vi "WSVCAP SHL Host LL I2C Read.vi"(0 "Bytes to Read":u8=8, 1 "Wait Ticks":u32, 2 "Slave Address":u8, 5 "Sub Address [U8]":u8=191 format="%.0x", 7 "Socket Mask [U64]":u64=1 format="%012x", 11 "error in":errorcluster, 12 "UUT Set (0/1)":u8) -> (4 "C1:1-18 Read Data [DUT Ordered]":u8[][](array[numeric]), 6 "C2:1-18 Read Data [DUT Ordered]":u8[][](array[numeric]), 8 "C3:1-18 Read Data [DUT Ordered]":u8[][](array[numeric]), 10 "Status":u8[](array[numeric]) format="%.0x", 15 "error out":errorcluster)   [LabVIEW 2012]
uses:
  Type Defs/WSVCAP SHL Top Level Write Read State Enum.ctl
  Type Defs/WSVCAP SHL State.ctl
  Type Defs/WSVCAP SHL Transaction Enum.ctl
  Type Defs/WSVCAP SHL Top Level Control Enum.ctl
panel:
  out "Bit Array":u64[](array[numeric]) format="%.0x"
  out "Data Headers":u8[](array[numeric])=[1, 2, 3, 4, 5, 6, 7, 8, 9, 10, 11, 12, 12, 14, 15, 16]
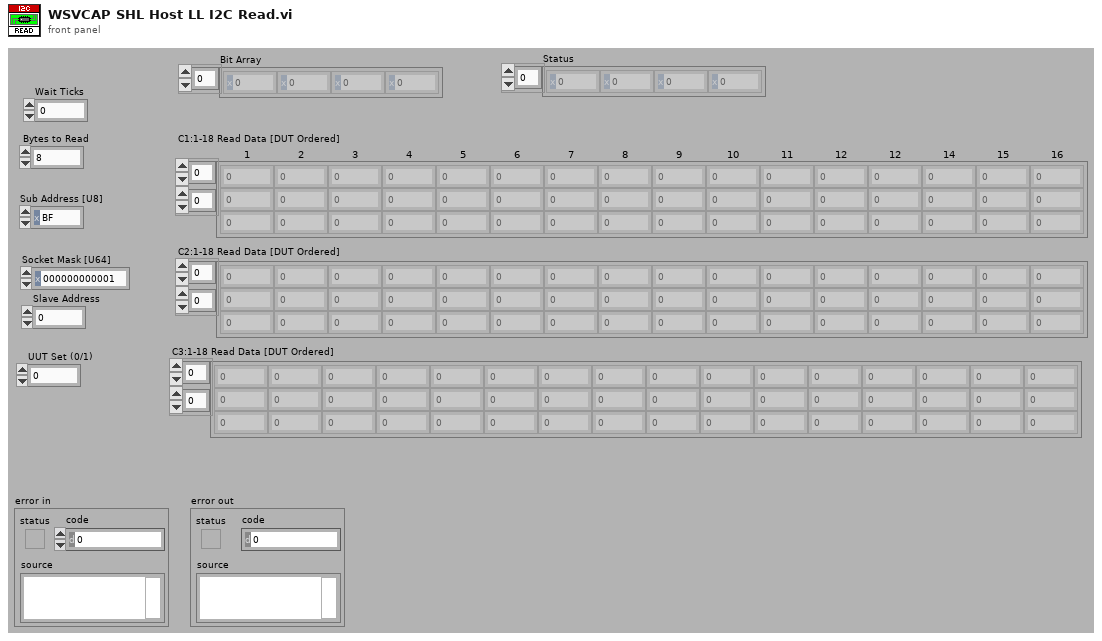
[diagram p1: front panel]
types:
  T1 = typedef "WSVCAP SHL Top Level Write Read State Enum.ctl" = enum16{"Start", "Write", "Read", "Get Status", "Wait Until Done"}
  T2 = typedef "WSVCAP SHL Transaction Enum.ctl" = enum16{"I2C-Read Data", "I2C-Write Data", "RFFE-Ext Write", "RFFE-Ext Read"}
  T3 = typedef "WSVCAP SHL Top Level Control Enum.ctl" = enum16{"Start", "Cmd", "Transaction", "Wait Ticks", "Socket Mask", "UUT Set", "Slave Address", "Sub Address", "Bytes to Write", "Bytes to Read", "Write Data", "Write Flag", "Read Data", "Read Flag", "Ack Read", "Read Status Flag", "Ack Read Status", "Status", "Cycle Count", "Stop Cycle", "Exit"}
  T4 = typedef "WSVCAP SHL State.ctl" = enum8{"Idle", "Transfer Data"}
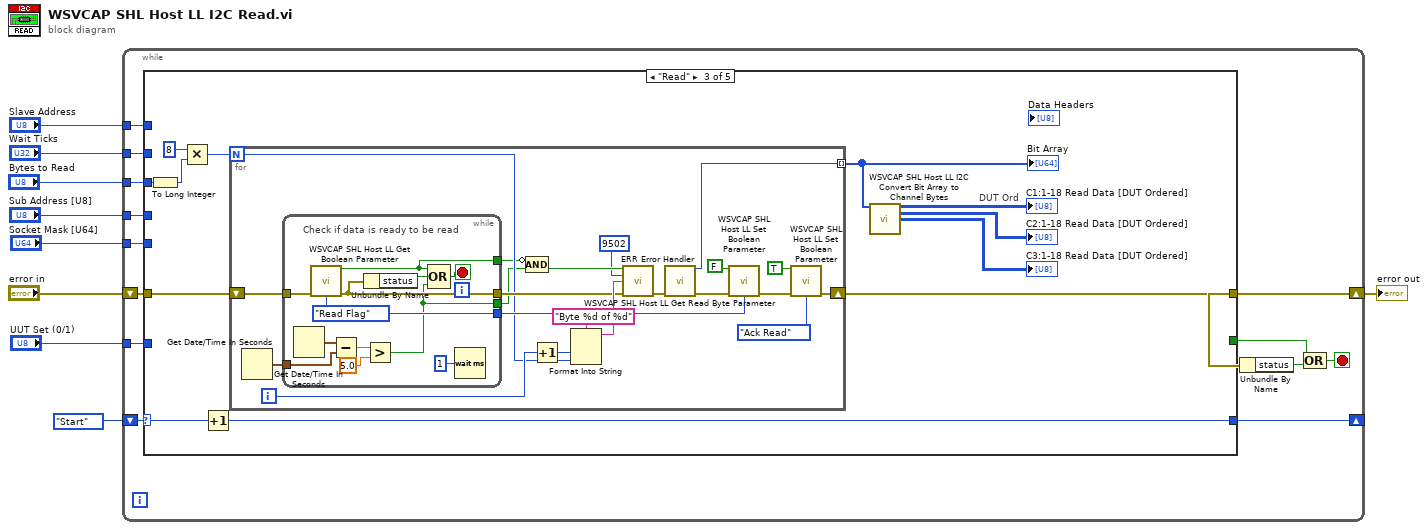
[diagram p0: block diagram]
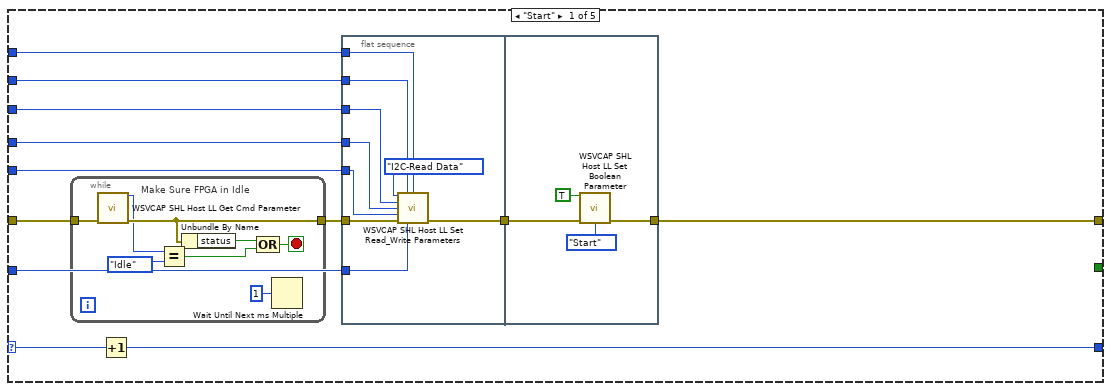
[diagram p2: hidden frame]
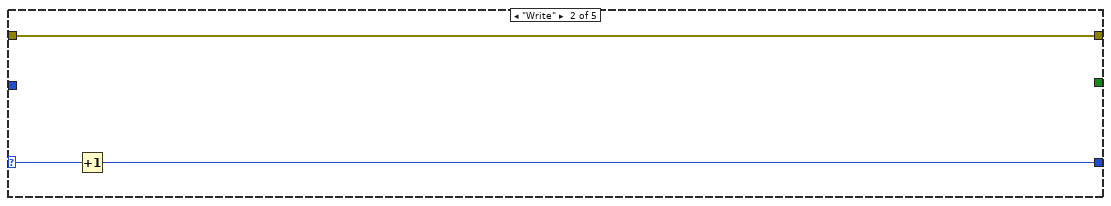
[diagram p3: hidden frame]
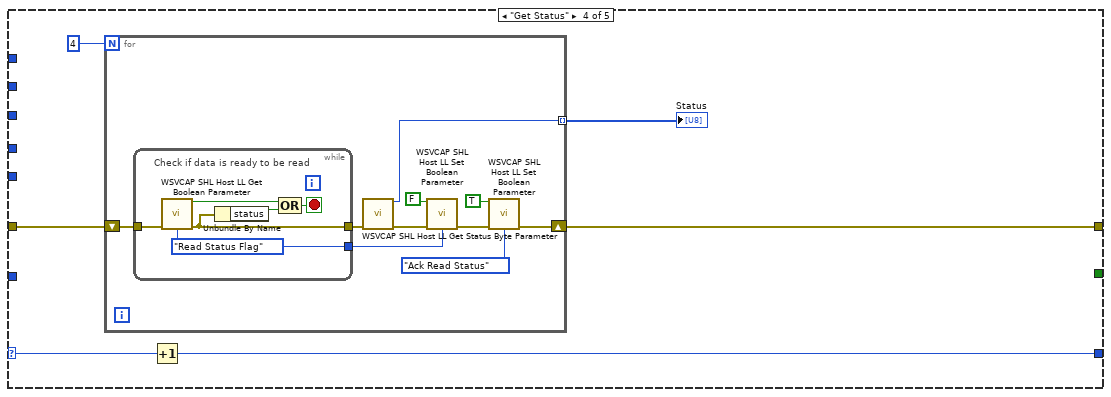
[diagram p4: hidden frame]
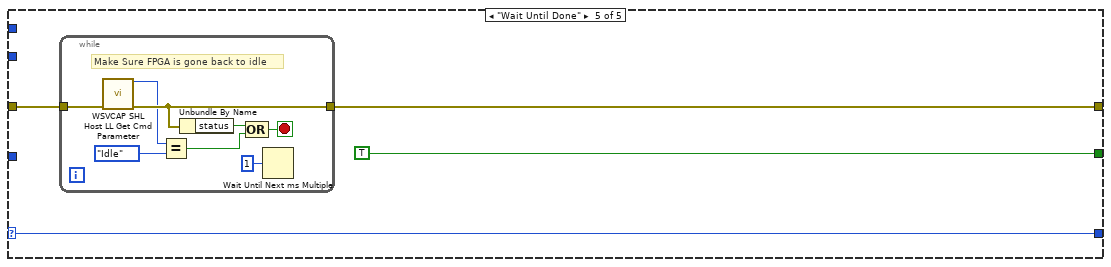
[diagram p5: hidden frame]
diagram:
  n1 = while {
    shift-right: [w21] -> w8
    shift-left: "error in" -> [w22]
    shift-right: [w16] -> _
    shift-left: WSVCAP_SHL_Top_Level_Write_Read_State_Enum."Start" ("Write Read State") -> [w17]
    tunnel: "Bytes to Read" -> [w15]
    tunnel: "Sub Address [U8]" -> [w14]
    tunnel: "Socket Mask [U64]" -> [w13]
    tunnel: "Wait Ticks" -> [w12]
    tunnel: "Slave Address" -> [w11]
    tunnel: "UUT Set (0/1)" -> [w10]
    stop <- w18 stop-if-true
    n2 = case shown="\"Read\"" w17 {
      selector: w17 -> [w33 w56 w68 w106 w126]
      tunnel: w22 -> [w34 w55 w61 w108 w128]
      tunnel: [w29 w55 w69 w107 w127] -> w21
      tunnel: [_ _ _ _ TRUE] -> w20
      tunnel: [w32 w57 w67 w105 w126] -> w16
      tunnel: w15 -> [w31 _ w66 _ _]
      tunnel: w14 -> [w27 _ _ _ _]
      tunnel: w13 -> [w26 _ _ _ _]
      tunnel: w12 -> [w25 _ _ _ _]
      tunnel: w11 -> [w24 _ _ _ _]
      tunnel: w10 -> [w23 _ _ _ _]
      frame "Start" {
        n3 = while {
          tunnel: w34 -> [w50]
          tunnel: [w49] -> w30
          stop <- w54 stop-if-true
          # "Make Sure FPGA in Idle"
          n4 = call "WSVCAP SHL Host LL Get Cmd Parameter.vi"("error in (no error)"=w50) -> ("I2C_Cmd"=w48:T4, "error out"=w49:errorcluster)  [unwired: 13 in]
          n5 = Equal?(x=w48, y=WSVCAP_SHL_State."Idle" ("Type")) -> (x = y?=w52:bool)
          n6 = Unbundle By Name(w49) -> ("status"=w47:bool)
          n7 = Compound Arithmetic op=OR(w47, w52) -> (w54:bool)
          n8 = Wait Until Next ms Multiple(millisecond multiple=u32 1) -> ()  [unwired: 1 out]
        }
        n9 = Increment(x=w33) -> (x+1=w32:T1)
        n10 = flat-sequence {
          tunnel: w31 -> [w40]
          tunnel: w30 -> [w43]
          tunnel: [w41] -> w28
          tunnel: w27 -> [w38]
          tunnel: w26 -> [w39]
          tunnel: w25 -> [w37]
          tunnel: w24 -> [w36]
          tunnel: w23 -> [w35]
          tunnel: [w46] -> w29
          tunnel: w28 -> [w46]
          frame #0 {
            n11 = call "WSVCAP SHL Host LL Set Read_Write Parameters.vi"("Transaction"=WSVCAP_SHL_Transaction_Enum."I2C-Read Data", "Wait Ticks"=w37, "Slave Address"=w36, "Bytes"=w40, "Sub Address [U8]"=w38, "Socket Mask [U64]"=w39, "error in (no error)"=w43, "UUT Set (0/1)"=w35) -> ("error out"=w41:errorcluster)  [unwired: 7 in]
          }
          frame #1 {
            n12 = call "WSVCAP SHL Host LL Set Boolean Parameter.vi"("Boolean In"=TRUE, "error in (no error)"=w46, "FPGA Top Level Control"=WSVCAP_SHL_Top_Level_Control_Enum."Start") -> ()  [unwired: 12 in, 1 out]
          }
        }
      }
      frame "Write" {
        n13 = Increment(x=w56) -> (x+1=w57:T1)
      }
      frame "Read" {
        # "DUT Ord"
        n14 = To Long Integer(number=w66) -> (32bit integer=w65:i32)
        n15 = Multiply(x=8, y=w65) -> (x*y=w63:i32)
        n16 = Increment(x=w68) -> (x+1=w67:T1)
        n17 = for {
          N: w63 -> [w73]
          shift-right: [w88] -> w69
          shift-left: w61 -> [w90]
          tunnel: [w82] -> w64 mode=indexing
          i -> [w74]
          n18 = Get Date/Time In Seconds() -> (seconds since 1Jan1904=w70:timestamp)
          n19 = while {
            tunnel: w90 -> [w101]
            tunnel: [w100] -> w76
            tunnel: [w98] -> w87
            tunnel: w70 -> [w95]
            tunnel: [w92] -> w72
            tunnel: [w91] -> w71
            stop <- w102 stop-if-true
            w98 = WSVCAP_SHL_Top_Level_Control_Enum."Read Flag" ("FPGA Top Level Control")
            # "Check if data is ready to be read"
            n20 = Get Date/Time In Seconds() -> (seconds since 1Jan1904=w96:timestamp)
            n21 = call "WSVCAP SHL Host LL Get Boolean Parameter.vi"("error in (no error)"=w101, "FPGA Top Level Control"=w98) -> ("Boolean Out"=w92:bool, "error out"=w100:errorcluster)  [unwired: 12 in]
            n22 = Subtract(x=w96, y=w95) -> (x-y=w94:dbl)
            n23 = Unbundle By Name(w100) -> ("status"=w99:bool)
            n24 = Greater?(x=w94, y=5.0) -> (0:w91:bool)
            n25 = Compound Arithmetic op=OR(w92, w99, w91) -> (w102:bool)
            n26 = Wait (ms)(milliseconds to wait=u32 1) -> ()  [unwired: 1 out]
          }
          n27 = Compound Arithmetic op=AND(invert w72, w71) -> (w81:bool)
          n28 = Increment(x=w74) -> (x+1=w77:i32)
          n29 = Format Into String(format string="Byte %d of %d", w77, w73) -> (resulting string=w79:string)  [unwired: 2 in, 1 out]
          n30 = call "ERR Error Handler.vi"("Error Status"=w81, "Error Code"=9502, "Cause Of Error"=w79, "Error In (no error)"=w76) -> ("Error Out"=w75:errorcluster)  [unwired: 11 in]
          n31 = call "WSVCAP SHL Host LL Get Read Byte Parameter.vi"("error in (no error)"=w75) -> ("Read Data In"=w82:u64, "error out"=w89:errorcluster)  [unwired: 13 in]
          n32 = call "WSVCAP SHL Host LL Set Boolean Parameter.vi"("Boolean In"=FALSE ("Read Flag"), "error in (no error)"=w89, "FPGA Top Level Control"=w87) -> ("error out"=w83:errorcluster)  [unwired: 12 in]
          n33 = call "WSVCAP SHL Host LL Set Boolean Parameter.vi"("Boolean In"=TRUE ("Write Flag"), "error in (no error)"=w83, "FPGA Top Level Control"=WSVCAP_SHL_Top_Level_Control_Enum."Ack Read") -> ("error out"=w88:errorcluster)  [unwired: 12 in]
        }
        "Bit Array" <- w64
        n34 = call "WSVCAP SHL Host LL I2C Convert Bit Array to Channel Bytes.vi"("Bit Array"=w64) -> ("C1:1-18 Read Data [SKT Ordered]"=→"C1:1-18 Read Data [DUT Ordered]":u8[][], "C2:1-18 Read Data [SKT Ordered]"=→"C2:1-18 Read Data [DUT Ordered]":u8[][], "C3:1-18 Read Data [SKT Ordered]"=→"C3:1-18 Read Data [DUT Ordered]":u8[][])  [unwired: 12 in]
      }
      frame "Get Status" {
        n35 = for {
          N: 4 -> [_]
          shift-right: [w115] -> w107
          shift-left: w108 -> [w118]
          tunnel: [w109] -> w104 mode=indexing
          n36 = while {
            tunnel: w118 -> [w122]
            tunnel: [w121] -> w117
            tunnel: [w119] -> w114
            stop <- w124 stop-if-true
            w119 = WSVCAP_SHL_Top_Level_Control_Enum."Read Status Flag" ("FPGA Top Level Control")
            # "Check if data is ready to be read"
            n37 = call "WSVCAP SHL Host LL Get Boolean Parameter.vi"("error in (no error)"=w122, "FPGA Top Level Control"=w119) -> ("Boolean Out"=w123:bool, "error out"=w121:errorcluster)  [unwired: 12 in]
            n38 = Unbundle By Name(w121) -> ("status"=w120:bool)
            n39 = Compound Arithmetic op=OR(w123, w120) -> (w124:bool)
          }
          n40 = call "WSVCAP SHL Host LL Get Status Byte Parameter.vi"("error in (no error)"=w117) -> ("I2C Status Byte"=w109:u8, "error out"=w116:errorcluster)  [unwired: 13 in]
          n41 = call "WSVCAP SHL Host LL Set Boolean Parameter.vi"("Boolean In"=FALSE ("Read Flag"), "error in (no error)"=w116, "FPGA Top Level Control"=w114) -> ("error out"=w110:errorcluster)  [unwired: 12 in]
          n42 = call "WSVCAP SHL Host LL Set Boolean Parameter.vi"("Boolean In"=TRUE ("Write Flag"), "error in (no error)"=w110, "FPGA Top Level Control"=WSVCAP_SHL_Top_Level_Control_Enum."Ack Read Status") -> ("error out"=w115:errorcluster)  [unwired: 12 in]
        }
        "Status" <- w104
        n43 = Increment(x=w106) -> (x+1=w105:T1)
      }
      frame "Wait Until Done" {
        n44 = while {
          tunnel: w128 -> [w131]
          tunnel: [w130] -> w127
          stop <- w133 stop-if-true
          # "Make Sure FPGA is gone back to idle"
          n45 = call "WSVCAP SHL Host LL Get Cmd Parameter.vi"("error in (no error)"=w131) -> ("I2C_Cmd"=w129:T4, "error out"=w130:errorcluster)  [unwired: 13 in]
          n46 = Equal?(x=w129, y=WSVCAP_SHL_State."Idle") -> (x = y?=w134:bool)
          n47 = Unbundle By Name(w130) -> ("status"=w135:bool)
          n48 = Compound Arithmetic op=OR(w135, w134) -> (w133:bool)
          n49 = Wait Until Next ms Multiple(millisecond multiple=u32 1) -> ()  [unwired: 1 out]
        }
      }
    }
    n50 = Unbundle By Name(w21) -> ("status"=w19:bool)
    n51 = Compound Arithmetic op=OR(w20, w19) -> (w18:bool)
  }
  "error out" <- w8
